vi "Set Boolean.vi"(7 "Name":string="Set Boolean", 10 "Boolean Value":bool, 11 "Abs_Boolean.lvclass":refnum<class "Abs_Boolean.lvclass">) -> (3 "Node":refnum<class "abs_Node.lvclass">)   [LabVIEW 2021, in "BT.lvlib"]
uses:
  BT.lvlib
  Set Boolean/Set Boolean.lvclass
  LV_Abstract/Source/Abs_Types/Boolean/Abs_Boolean.lvclass
  C:/Users/Tim/Documents/GitHub/LV_Abstract/Source/Abs_Types/Value/Abs_Value.lvclass
  C:/Users/Tim/Documents/GitHub/LV_Abstract/Source/Abs_Types/Type/Abs_Type.lvclass
  C:/Users/Tim/Documents/GitHub/LV_Abstract/Source/Abs_Types/Boolean/Abs_Boolean.lvclass
  C:/Users/Tim/Documents/LabVIEW/2021/Behaviour Tree/Source/abs_Type Leaf/abs_Type Leaf.lvclass
  C:/Users/Tim/Documents/LabVIEW/2021/Behaviour Tree/Source/abs_Leaf/abs_Leaf.lvclass
  C:/Users/Tim/Documents/LabVIEW/2021/Behaviour Tree/Source/abs_Node/abs_Node.lvclass
  C:/Users/Tim/Documents/LabVIEW/2021/Behaviour Tree/Source/Set Boolean/Set Boolean.lvclass
  abs_Node/abs_Node.lvclass
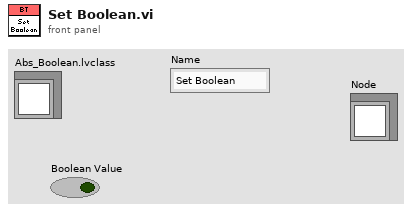
[diagram p1: front panel]
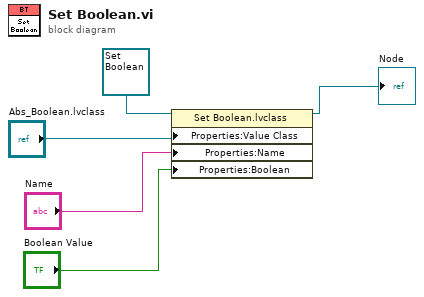
[diagram p0: block diagram]
diagram:
  n1 = property class="Set Boolean.lvclass"(reference=refnum<class "Set Boolean.lvclass"> refnum ("BT.lvlib:Set Boolean.lvclass"), "Properties:Value Class"="Abs_Boolean.lvclass", "Properties:Name"="Name", "Properties:Boolean"="Boolean Value") -> (reference out=→"Node":refnum<class "Set Boolean.lvclass">)  [unwired: 1 in, 1 out]
